vi "Write_Spreadsheet.vi"(0 "File_Path_In":path, 7 "Table":string[][](array[string]), 11 "Error_In":errorcluster) -> (4 "File_Path_Out":path, 15 "Error_Out":errorcluster)   [LabVIEW 2023, in "File_Handler_Library.lvlib"]
doc: "This VI Writes the given data to CSV file"
uses:
  File_Handler_Library.lvlib
  Library_Controls/Mode.ctl
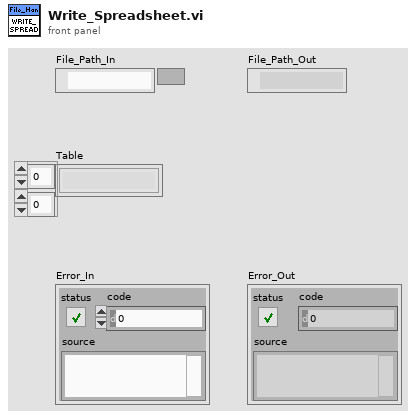
[diagram p1: front panel]
types:
  T1 = typedef "File_Handler_Library.lvlib/Mode.ctl" = enum16{"Write", "Read"}
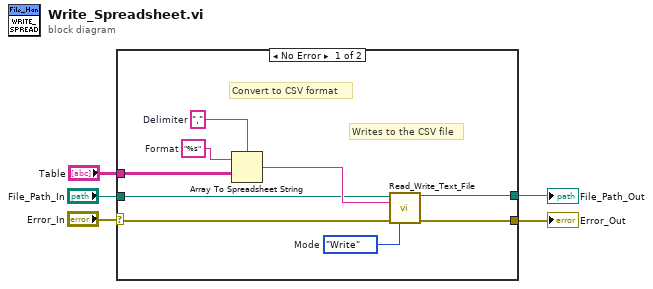
[diagram p0: block diagram]
diagram:
  n1 = case shown="No Error" "Error_In" {
    selector: "Error_In" -> [w11 w16]
    tunnel: [w12 w16] -> w5
    tunnel: "File_Path_In" -> [w8 w15]
    tunnel: [w7 w15] -> w2
    tunnel: "Table" -> [w6 _]
    frame No Error {
      w9 = Mode."Write"  # Mode
      w13 = "%s"  # Format
      w14 = ","  # Delimiter
      # "Convert to CSV format"
      # "Writes to the CSV file"
      n2 = Array To Spreadsheet String(delimiter (Tab)=w14, array=w6, 3:w13) -> (spreadsheet string=w10:string)
      n3 = call "Read_Write_Text_File.vi"("File_Path_In"=w8, "Data_In"=w10, "Error_In"=w11, "Mode"=w9) -> ("File_Path_Out"=w7:path, "Error_Out"=w12:errorcluster)  [unwired: 9 in, 1 out]
    }
    frame Error {
    }
  }
  "Error_Out" <- w5
  "File_Path_Out" <- w2
